vi "SUB_COM_W_CharByCharNoCarrige_HEX.vi"(2 "cmd string":string, 3 "duplicate VISA resource name":refnum<visa-resource-name>) -> (0 "OUT string":string, 1 "VISA resource OUT":refnum<visa-resource-name>)   [LabVIEW 2011]
panel:
  out "out1":string
  out "LOOP":i32
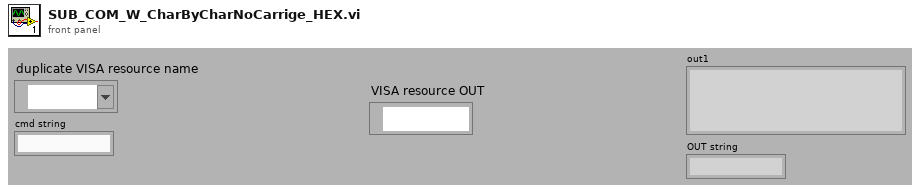
[diagram p1: front panel]
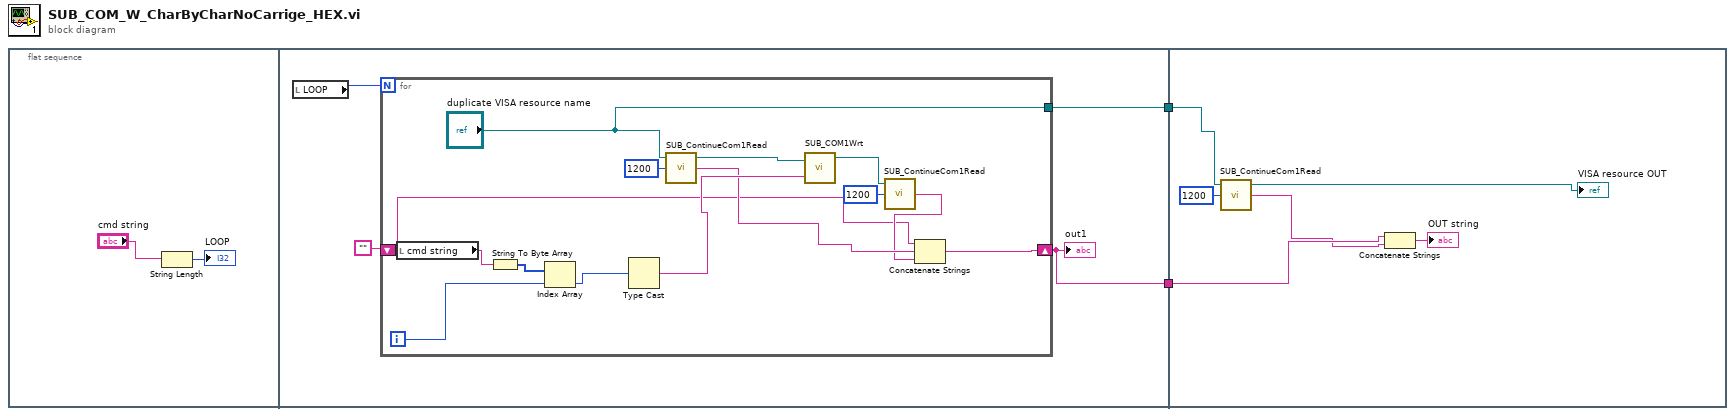
[diagram p0: block diagram]
diagram:
  n1 = flat-sequence {
    tunnel: [w7] -> w2
    tunnel: [w5] -> w1
    tunnel: w2 -> [w27]
    tunnel: w1 -> [w25]
    frame #0 {
      n2 = String Length(string="cmd string") -> (length=→"LOOP":i32)
    }
    frame #1 {
      n3 = local read "LOOP"() -> (w8:i32)
      n4 = for {
        N: w8 -> [_]
        tunnel: ["duplicate VISA resource name"] -> w7
        shift-right: [w10] -> w5
        shift-left: "" -> [w9]
        i -> [w16]
        n5 = local read "cmd string"() -> (w18:string)
        n6 = String To Byte Array(string=w18) -> (unsigned byte array=w17:u8[])
        n7 = Index Array(array=w17, index=w16) -> (element=w15:u8)
        n8 = Type Cast(x=w15) -> (*(type *) &x=w14:string)  [unwired: 1 in]
        n9 = call "SUB_ContinueCom1Read.vi"("Numeric"=1200, "duplicate VISA resource name 2"="duplicate VISA resource name") -> ("String"=w12:string, "duplicate VISA resource name"=w19:refnum<visa-resource-name>)  [unwired: 1 in, 1 out]
        n10 = call "SUB_COM1Wrt.vi"("VISA resource name"=w19, "write buffer"=w14) -> ("duplicate VISA resource name"=w21:refnum<visa-resource-name>)  [unwired: 2 out]
        n11 = call "SUB_ContinueCom1Read.vi"("Numeric"=1200, "duplicate VISA resource name 2"=w21) -> ("String"=w11:string)  [unwired: 1 in, 2 out]
        n12 = Concatenate Strings(w9, w12, w11) -> (w10:string)
      }
      "out1" <- w5
    }
    frame #2 {
      n13 = call "SUB_ContinueCom1Read.vi"("Numeric"=1200, "duplicate VISA resource name 2"=w27) -> ("String"=w24:string, "duplicate VISA resource name"=→"VISA resource OUT":refnum<visa-resource-name>)  [unwired: 1 in, 1 out]
      n14 = Concatenate Strings(w25, w24) -> (→"OUT string":string)
    }
  }
